vi "CoboltLaser_Example_LaserStatusBasicGet.vi"(0 "ComPort":refnum<visa-resource-name>, 7 "error in (no error)":errorcluster) -> (27 "error out":errorcluster)   [LabVIEW 2019]
panel:
  out "OperatingHours":dbl
  out "Fault":string
  out "LaserOn":bool
  out "SerialNumber":string
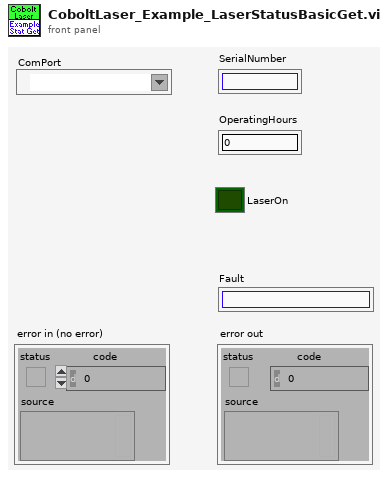
[diagram p1: front panel]
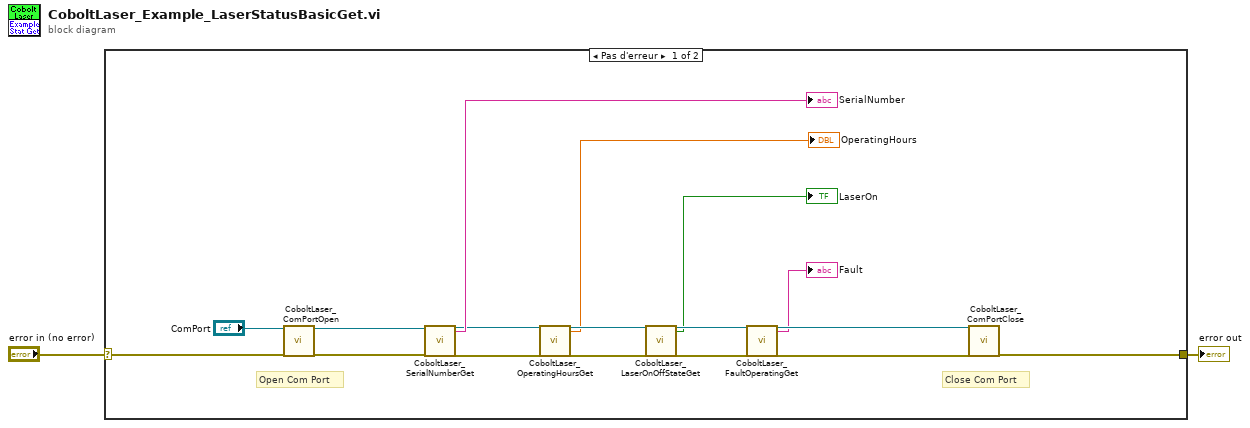
[diagram p0: block diagram]
diagram:
  n1 = case shown="Pas d'erreur" "error in (no error)" {
    selector: "error in (no error)" -> [w19 w20]
    tunnel: [w15 w20] -> w1
    frame No Error {
      # "Close Com Port"
      # "Open Com Port"
      n2 = call <userlib>:"CoboltLaser_ComPortOpen.vi"("ComPort"="ComPort", "error in (no error)"=w19) -> ("ComPort Out"=w13:refnum<visa-resource-name>, "error out"=w18:errorcluster)  [unwired: 16 in]
      n3 = call <userlib>:"CoboltLaser_SerialNumberGet.vi"("ComPort"=w13, "error in (no error)"=w18) -> ("ComPortOut"=w6:refnum<visa-resource-name>, "SerialNumber"=→"SerialNumber":string, "error out"=w8:errorcluster)  [unwired: 22 in, 1 out]
      n4 = call <userlib>:"CoboltLaser_OperatingHoursGet.vi"("ComPort"=w6, "error in (no error)"=w8) -> ("ComPortOut"=w5:refnum<visa-resource-name>, "OperatingHours"=→"OperatingHours":dbl, "error out"=w7:errorcluster)  [unwired: 23 in]
      n5 = call <userlib>:"CoboltLaser_LaserOnOffStateGet.vi"("ComPort"=w5, "error in (no error)"=w7) -> ("ComPortOut"=w12:refnum<visa-resource-name>, "On"=→"LaserOn":bool, "error out"=w17:errorcluster)  [unwired: 21 in, 2 out]
      n6 = call <userlib>:"CoboltLaser_FaultOperatingGet.vi"("ComPort"=w12, "error in (no error)"=w17) -> ("ComPortOut"=w11:refnum<visa-resource-name>, "Fault"=→"Fault":string, "error out"=w16:errorcluster)  [unwired: 23 in]
      n7 = call <userlib>:"CoboltLaser_ComPortClose.vi"("ComPort"=w11, "error in (no error)"=w16) -> ("error out"=w15:errorcluster)  [unwired: 17 in]
    }
    frame Error {
    }
  }
  "error out" <- w1
